vi "apply modification.vi"(10 "vis":refnum<vi>[](array[refnum]), 11 "set source separate in":refnum<class "set source separate.lvclass">) -> (0 "error report":errorcluster[](array[cluster]), 3 "set source separate out":refnum<class "set source separate.lvclass">)   [LabVIEW 2013, in "set source separate.lvclass"]
uses:
  set source separate.lvclass
  set source separate.lvclass/set source separate.ctl
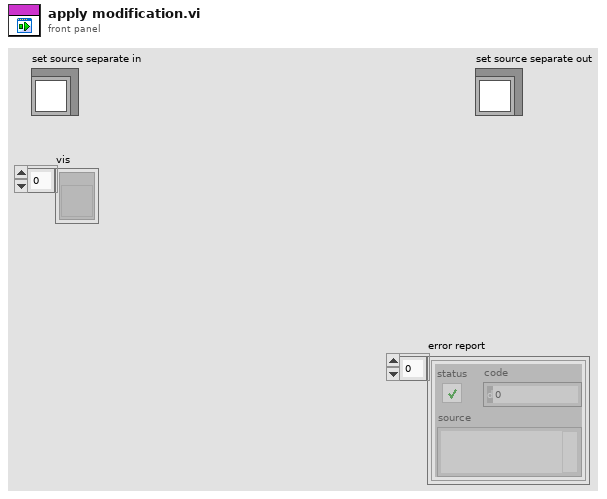
[diagram p1: front panel]
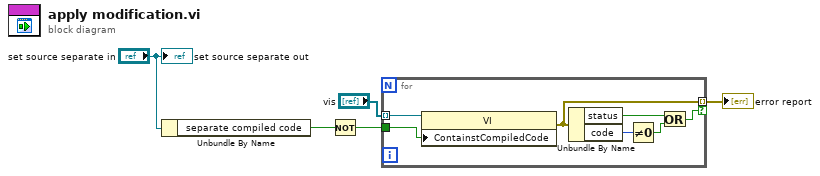
[diagram p0: block diagram]
diagram:
  n1 = Unbundle By Name("set source separate in") -> ("separate compiled code"=w2:bool)
  n2 = Not(x=w2) -> (.not. x?=w1:bool)
  n3 = for {
    tunnel: "vis" -> [w12] mode=indexing
    tunnel: [w8] -> w4 mode=indexing if=w7
    tunnel: w1 -> [w6]
    n4 = property class="VI"(reference=w12, "ContainstCompiledCode"=w6) -> (error out=w8:errorcluster)  [unwired: 1 in, 1 out]
    n5 = Unbundle By Name(w8) -> ("status"=w11:bool, "code"=w10:i32)
    n6 = Not Equal To 0?(x=w10) -> (x != 0?=w9:bool)
    n7 = Or(x=w11, y=w9) -> (x .or. y?=w7:bool)
  }
  "error report" <- w4
  "set source separate out" <- "set source separate in"
